vi "Error.Check NoRetry Config.vi"(9 "Fault Code":i32, 11 "ConfigDir":path) -> (3 "NoRetry":bool)   [LabVIEW 2024, in "EQMF.lvlib" / "Errors.lvlib"]
uses:
  Errors.lvlib
  <vilib>/KATE/Files/File Utils.lvlib
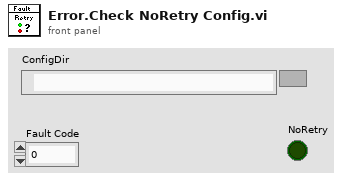
[diagram p1: front panel]
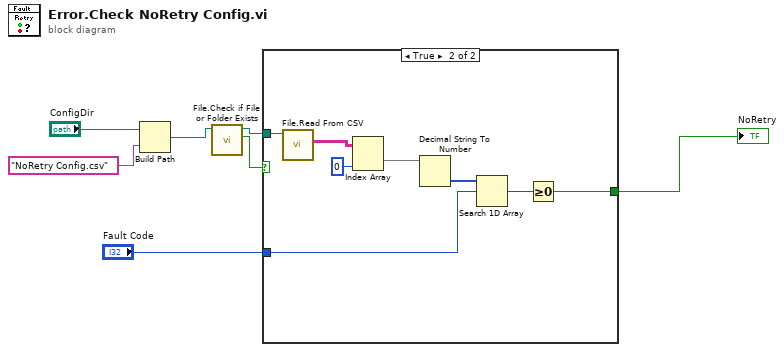
[diagram p0: block diagram]
diagram:
  n1 = Build Path(base path="ConfigDir", name or relative path="NoRetry Config.csv") -> (appended path=w3:path)
  n2 = call <vilib>:"File.Check if File or Folder Exists.vi"("Path"=w3) -> ("Exists"=w1:bool, "Dup Path"=w2:path)  [unwired: 6 in, 3 out]
  n3 = case shown="True" w1 {
    tunnel: "Fault Code" -> [_ w11]
    tunnel: [_ w9] -> w4
    tunnel: w2 -> [_ w8]
    frame False {
    }
    frame True {
      n4 = call <vilib>:"File.Read From CSV.vi"("File"=w8) -> ("Data"=w15:string[][])  [unwired: 8 in, 2 out]
      n5 = Index Array(array=w15, index (col)=0 ("disabled index (col)")) -> (element=w13:string[])  [unwired: 1 in]
      n6 = Decimal String To Number(string=w13) -> (number=w12:i32[])  [unwired: 2 in, 1 out]
      n7 = Search 1D Array(1D array=w12, element=w11) -> (index of element=w10:i32)  [unwired: 1 in]
      n8 = Greater Or Equal To 0?(x=w10) -> (x >= 0?=w9:bool)
    }
  }
  "NoRetry" <- w4
